vi "Rectangle Comparison.vi"(9 "Second":dbl[](array[numeric]), 11 "First":dbl[](array[numeric])) -> (0 "Rect":T1, 3 "Scores":T2)   [LabVIEW 2017]
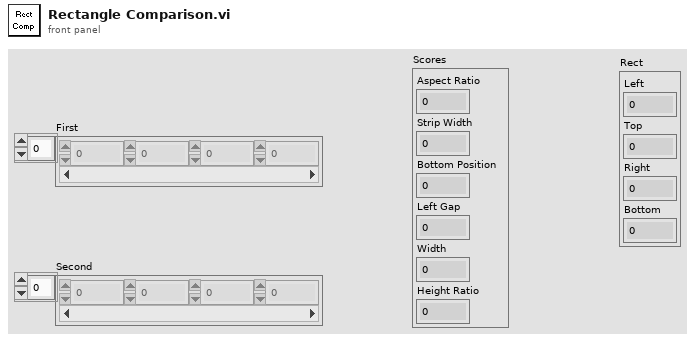
[diagram p1: front panel]
types:
  T1 = cluster{"Left":dbl, "Top":dbl, "Right":dbl, "Bottom":dbl}
  T2 = cluster{"Aspect Ratio":dbl, "Strip Width":dbl, "Bottom Position":dbl, "Left Gap":dbl, "Width":dbl, "Height Ratio":dbl}
  T3 = cluster{"[0]":dbl, "[1]":dbl, "[2]":dbl, "[3]":dbl}
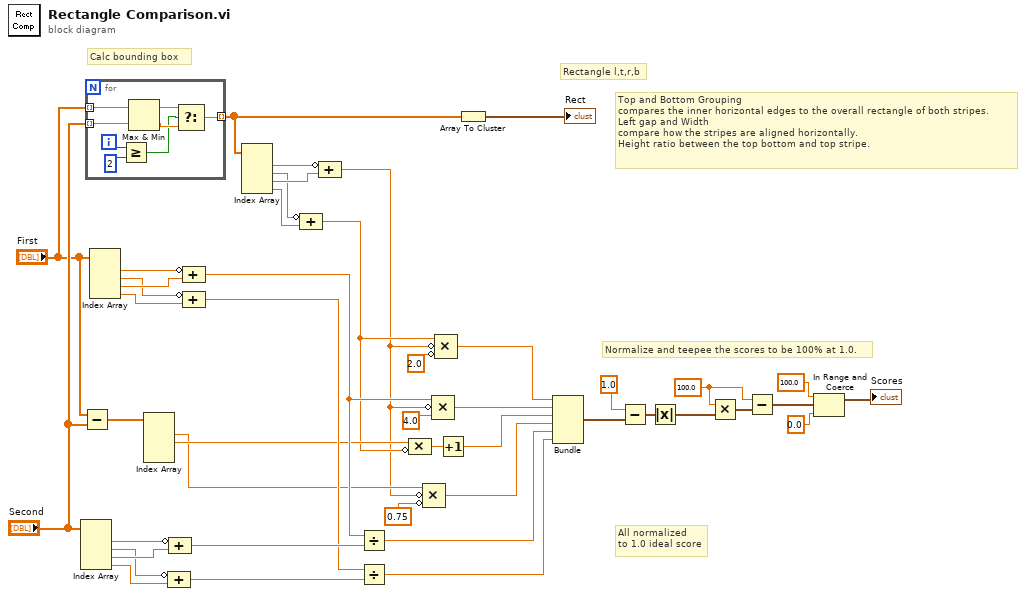
[diagram p0: block diagram]
diagram:
  w32 = 100.0 ("x/y")
  # "All normalized\nto 1.0 ideal score"
  # "Normalize and teepee the scores to be 100% at 1.0."
  # "Top and Bottom Grouping\ncompares the inner horizontal edges to the overall rectangle of both stripes.\nLeft gap and Width\ncompare how the stripes are aligned horizontally.\nHeight ratio between the top bottom and top stripe."
  # "Calc bounding box"
  # "Rectangle l,t,r,b"
  n1 = Index Array(array="Second") -> (element #1=w42:dbl, element #2=w23:dbl, element #3=w45:dbl, element #4=w7:dbl)  [unwired: 4 in]
  n2 = Subtract(x="First", y="Second") -> (x-y=w14:dbl[])
  n3 = for {
    tunnel: "First" -> [w53] mode=indexing
    tunnel: "Second" -> [w52] mode=indexing
    tunnel: [w46] -> w17 mode=indexing
    i -> [w50]
    n4 = Greater Or Equal?(x=w50, y=2) -> (x >= y?=w47:bool)
    n5 = Max & Min(x=w53, y=w52) -> (max(x,y)=w49:dbl, min(x,y)=w48:dbl)
    n6 = Select(t=w49, s=w47, f=w48) -> (s? t:f=w46:dbl)
  }
  n7 = Index Array(array="First") -> (element #1=w37:dbl, element #2=w22:dbl, element #3=w36:dbl, element #4=w38:dbl)  [unwired: 4 in]
  n8 = Index Array(array=w14) -> (element #1=w12:dbl, element #2=w13:dbl)  [unwired: 4 in, 2 out]
  n9 = Compound Arithmetic op=ADD(invert w23, w7) -> (w43:dbl)
  n10 = Compound Arithmetic op=ADD(invert w42, w45) -> (w44:dbl)
  n11 = Compound Arithmetic op=ADD(invert w37, w36) -> (w20:dbl)
  n12 = Compound Arithmetic op=ADD(invert w22, w38) -> (w24:dbl)
  n13 = Index Array(array=w17) -> (element #1=w9:dbl, element #2=w6:dbl, element #3=w8:dbl, element #4=w5:dbl)  [unwired: 4 in]
  n14 = Compound Arithmetic op=ADD(invert w6, w5) -> (w4:dbl)
  n15 = Compound Arithmetic op=ADD(invert w9, w8) -> (w3:dbl)
  n16 = Divide(x=w20, y=w44) -> (x/y=w40:dbl)
  n17 = Divide(x=w24, y=w43) -> (x/y=w39:dbl)
  n18 = Compound Arithmetic op=MULTIPLY(w13, invert w4) -> (w19:dbl)
  n19 = Compound Arithmetic op=MULTIPLY(w12, invert w3, invert 0.75 ("y")) -> (w15:dbl)
  n20 = Compound Arithmetic op=MULTIPLY(w20, invert w3, 4.0 ("y")) -> (w41:dbl)
  n21 = Compound Arithmetic op=MULTIPLY(w4, invert w3, invert 2.0 ("y")) -> (w1:dbl)
  n22 = Increment(x=w19) -> (x+1=w18:dbl)
  n23 = Array To Cluster(array=w17) -> (cluster=→"Rect":T3)
  n24 = Bundle(w1, w41, w18, w15, w40, w39) -> (w26:cluster{dbl, dbl, dbl, dbl, dbl, dbl})  [unwired: 1 in]
  n25 = Subtract(x=1.0 ("y"), y=w26) -> (x-y=w30:cluster{dbl, dbl, dbl, dbl, dbl, dbl})
  n26 = Absolute Value(x=w30) -> (abs(x)=w33:cluster{dbl, dbl, dbl, dbl, dbl, dbl})
  n27 = Multiply(x=w32, y=w33) -> (x*y=w34:cluster{dbl, dbl, dbl, dbl, dbl, dbl})
  n28 = Subtract(x=w32, y=w34) -> (x-y=w29:cluster{dbl, dbl, dbl, dbl, dbl, dbl})
  n29 = In Range and Coerce(upper limit=100.0, x=w29, lower limit=0.0) -> (coerced(x)=→"Scores":cluster{dbl, dbl, dbl, dbl, dbl, dbl})  [unwired: 1 out]
